vi "Area.vi"(8 "error in (no error)":errorcluster, 11 "Collection in":refnum<class "Collection.lvclass">) -> (0 "error out":errorcluster, 2 "Area":T1, 3 "Collection out":refnum<class "Collection.lvclass">)   [LabVIEW 2021, in "Picture2D.lvlib" / "Collection.lvclass"]
uses:
  Collection.lvclass
  Collection.lvclass/Collection.ctl
  IDrawable/IDrawable.lvclass
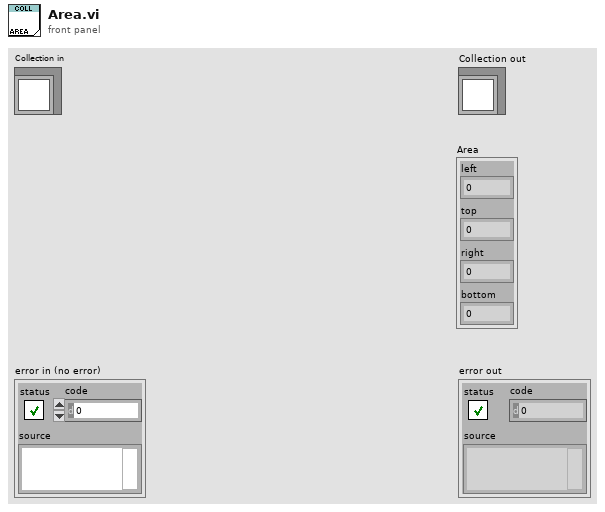
[diagram p1: front panel]
types:
  T1 = cluster{"left":i16, "top":i16, "right":i16, "bottom":i16}
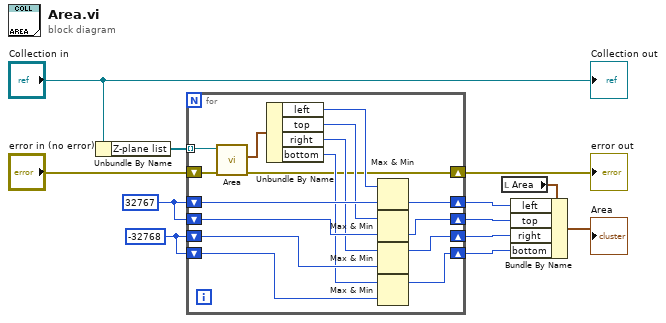
[diagram p0: block diagram]
diagram:
  w5 = i16 -32768
  w6 = i16 32767
  n1 = Unbundle By Name("Collection in") -> ("Z-plane list"=w11:refnum<class "IDrawable.lvclass">[])
  n2 = for {
    tunnel: w11 -> [w28] mode=indexing
    shift-right: [w24] -> w8
    shift-left: w6 -> [w25]
    shift-right: [w21] -> w4
    shift-left: w6 -> [w23]
    shift-right: [w19] -> w3
    shift-left: w5 -> [w18]
    shift-right: [w20] -> w7
    shift-left: w5 -> [w17]
    shift-right: [w13] -> w1
    shift-left: "error in (no error)" -> [w14]
    n3 = call-dynamic "Area.vi"("error in (no error)"=w14, "IDrawable in"=w28) -> ("error out"=w13:errorcluster, "Area"=w27:T1)  [unwired: 7 in, 1 out]
    n4 = Unbundle By Name(w27) -> ("left"=w26:i16, "top"=w22:i16, "right"=w16:i16, "bottom"=w15:i16)
    n5 = Max & Min(x=w26, y=w25) -> (min(x,y)=w24:i16)  [unwired: 1 out]
    n6 = Max & Min(x=w22, y=w23) -> (min(x,y)=w21:i16)  [unwired: 1 out]
    n7 = Max & Min(x=w16, y=w18) -> (max(x,y)=w19:i16)  [unwired: 1 out]
    n8 = Max & Min(x=w15, y=w17) -> (max(x,y)=w20:i16)  [unwired: 1 out]
  }
  "error out" <- w1
  n9 = local read "Area"() -> (w10:T1)
  n10 = Bundle By Name(cluster=w10, "left"=w8, "top"=w4, "right"=w3, "bottom"=w7) -> (→"Area":T1)
  "Collection out" <- "Collection in"
